vi "Init FPGA code.vi"(8 "error in (no error)":errorcluster, 11 "Device Ref in":T1 format="%.0x") -> (0 "Error out":errorcluster, 1 "DMA FIFO ref":refnum<k20>, 2 "Bitfile ref":refnum<k20>, 3 "Device Ref out":T1 format="%.0x")   [LabVIEW 2014, in "SLSC configuration Engine.lvlib"]
uses:
  SLSC configuration Engine.lvlib
  <vilib>/NI Veristand/Custom Device API/Custom Device Item Ref.ctl
  Shared/Type Defs/Device Settings.ctl
  <vilib>/NI/LVFPGA Adv Session Resources/OpenByNameSubVI.vi
  Shared/Constants.vi
  <vilib>/NI Veristand/Custom Device API/Get Item Property (Variant).vi
  <vilib>/FPGAPlugInAG/Dynamic/niLvFpga_Run_Dynamic.vi
  <vilib>/rvi/interface/common/dynamic/niFpgaEscapeDelimiterAndNull.vi
  <vilib>/Utility/error.llb/Error Cluster From Error Code.vi
  <vilib>/rvi/errors/niLvFpgaAdjustHostInterfaceError.vi
  <vilib>/rvi/interface/nirviMethod/nirviMethod.xnode
  <vilib>/NI/LVFPGA Adv Session Resources/OpenByName.xnode
  <vilib>/rvi/interface/nirviReadWriteControl/nirviReadWriteControl.xnode
  <vilib>/NI Veristand/Custom Device API/Custom Device API.lvlib
  Shared/SLSC configuration Shared.lvlib
  <vilib>/NI/LVFPGA Adv Session Resources/LVFPGAAdvSessionResources.lvlib
  NiFpgaLv.dll
  <vilib>/rvi/interface/Simulation/niFpgaSimulationCallBeginRW.vi
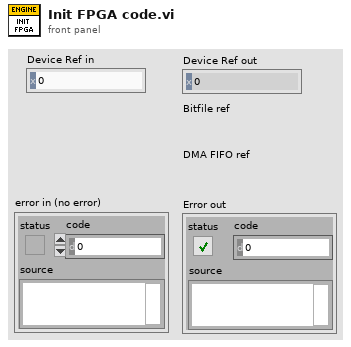
[diagram p1: front panel]
types:
  T1 = typedef "Custom Device API.lvlib/Custom Device Item Ref.ctl" = u64
  T2 = cluster{"Divide Value":u8, "Transfer Length (bits)":u8, "CS Asserted Polarity":bool, "Clock Polarity (CPOL)":bool, "Clock Phase (CPHA)":bool, "Lengthen MISO Setup":bool, "Direction Change Bit":u8, "MOSI Starts as Output":bool, "Tristatable MOSI":bool}
  T3 = typedef "SLSC configuration Shared.lvlib/Device Settings.ctl" = cluster{"RIO Address":string, "Bitfile Path":path, "Load Delay (ms)":u32, "Divide Value":u8, "Sample Rate (S/s)":u32}
  T4 = cluster{"Name":string, "Depth":u32, "Write? (Deprecated:Use Implementation)":bool, "Physical Channel":u32, "Base Address":u32, "Data Width":u32, "Data Type":enum32{"Boolean", "I8", "I16", "I32", "I64", "U8", "U16", "U32", "U64", "FXP", "CustomControl", "SGL"}, "FXP Properties":variant, "Write Window Address":u32, "Implementation":enum16{"niFpgaTargetToHost", "niFpgaHostToTarget", "niFpgaPeerToPeerWriter", "niFpgaPeerToPeerReader", "niCoreTargetToHost", "niCoreHostToTarget"}, "Control Set":u32}[]
  T5 = cluster{"Name":string, "type":variant, "indicator?":bool}[]
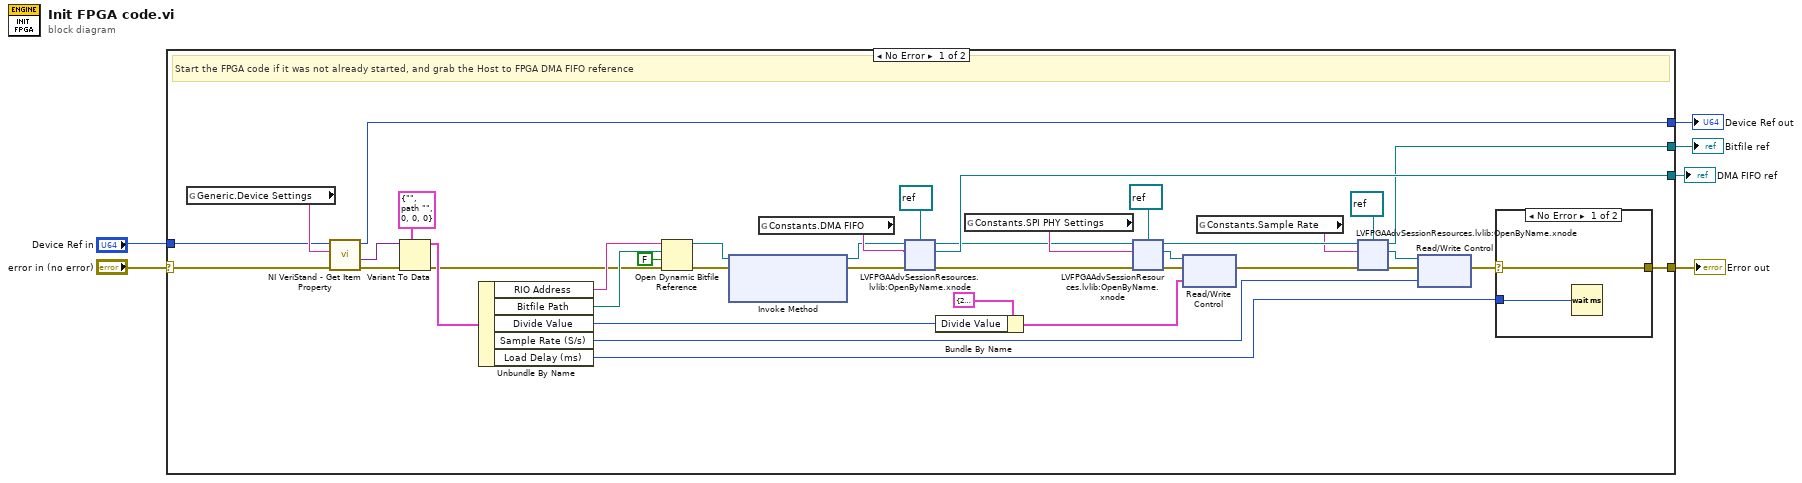
[diagram p0: block diagram]
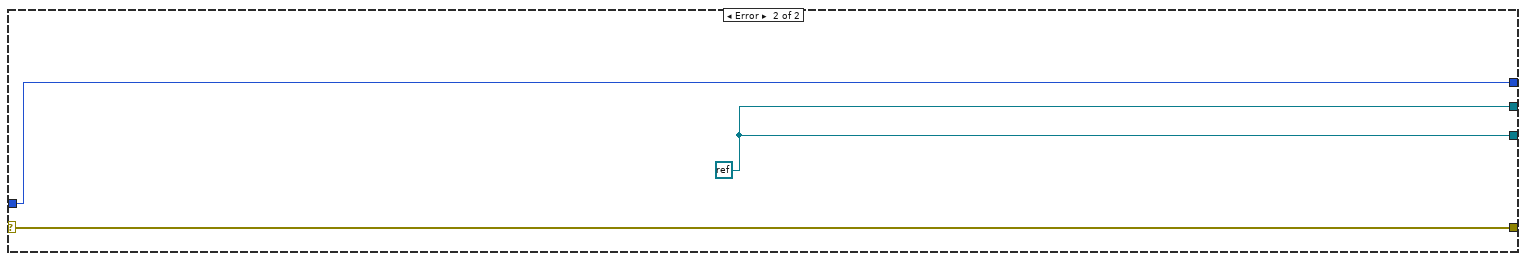
[diagram p3: hidden frame]
diagram:
  n1 = case shown="No Error" "error in (no error)" {
    selector: "error in (no error)" -> [w35 w89]
    tunnel: "Device Ref in" -> [w42 w88]
    tunnel: [w10 w90] -> w6
    tunnel: [w39 w90] -> w1
    tunnel: [w13 w89] -> w5
    tunnel: [w8 w88] -> w2
    frame No Error {
      # "Start the FPGA code if it was not already started, and grab the Host to FPGA DMA FIFO reference"
      n2 = global read "Constants.vi" "Generic.Device Settings"() -> (w43:string)
      n3 = call-poly <vilib>:"NI VeriStand - Get Item Property.vi"("error in (no error)"=w35, "Property Name"=w43, "Item Ref in"=w42) -> ("error out"=w33:errorcluster, "Value"=w34:variant, "Item Ref out"=w8:T1)  [unwired: 5 in, 1 out]
      n4 = Variant To Data(error in=w33, type=T3 {"RIO Address"="", "Bitfile Path"=path "", "Load Delay (ms)"=0, "Divide Value"=0, "Sample Rate (S/s)"=0} ("Cluster"), Variant=w34) -> (data=w31:T3, error out=w29:errorcluster)
      n5 = Unbundle By Name(w31) -> ("RIO Address"=w30:string, "Bitfile Path"=w44:path, "Divide Value"=w18:u8, "Sample Rate (S/s)"=w16:u32, "Load Delay (ms)"=w15:u32)
      n6 = Open Dynamic Bitfile Reference(0:w30, 1:w44, 2:FALSE ("Run When Loaded"), 3:w29) -> (5:w38:refnum<k20>, 8:w40:errorcluster)  [unwired: 1 in]
      n7 = xnode "Invoke Method"("FPGA VI Reference In"=w38, "error in"=w40) -> ("FPGA VI Reference Out"=w37:refnum<k20>, "error out"=w36:errorcluster)  [unwired: 1 in]
      n8 = global read "Constants.vi" "Constants.DMA FIFO"() -> (w41:string)
      n9 = xnode "LVFPGAAdvSessionResources.lvlib:OpenByName.xnode"("FPGA VI Reference in"=w37, "Resource name in"=w41, "Single resource reference type in"=refnum<k20> refnum ("Single resource reference out"), "Error in"=w36) -> ("Single resource reference out"=w39:refnum<k20>, "Error out"=w20:errorcluster, "FPGA VI Reference out"=w11:refnum<k20>)
      n10 = Bundle By Name(cluster=T2 {"Divide Value"=255, "Transfer Length (bits)"=32, "CS Asserted Polarity"=FALSE, "Clock Polarity (CPOL)"=FALSE, "Clock Phase (CPHA)"=FALSE, "Lengthen MISO Setup"=FALSE, "Direction Change Bit"=0, "MOSI Starts as Output"=FALSE, "Tristatable MOSI"=FALSE} ("SPI PHY Settings"), "Divide Value"=w18) -> (w17:T2)
      n11 = global read "Constants.vi" "Constants.SPI PHY Settings"() -> (w12:string)
      n12 = xnode "LVFPGAAdvSessionResources.lvlib:OpenByName.xnode"("FPGA VI Reference in"=w11, "Resource name in"=w12, "Single resource reference type in"=refnum<k20> refnum, "Error in"=w20) -> ("Single resource reference out"=w28:refnum<k20>, "Error out"=w27:errorcluster, "FPGA VI Reference out"=w25:refnum<k20>)
      n13 = xnode "Read/Write Control"("FPGA VI Reference In"=w28, "error in"=w27, "Value"=w17) -> ("error out"=w26:errorcluster)  [unwired: 1 out]
      n14 = global read "Constants.vi" "Constants.Sample Rate"() -> (w9:string)
      n15 = xnode "LVFPGAAdvSessionResources.lvlib:OpenByName.xnode"("FPGA VI Reference in"=w25, "Resource name in"=w9, "Single resource reference type in"=refnum<k20> refnum, "Error in"=w26) -> ("Single resource reference out"=w23:refnum<k20>, "Error out"=w24:errorcluster, "FPGA VI Reference out"=w10:refnum<k20>)
      n16 = xnode "Read/Write Control"("FPGA VI Reference In"=w23, "error in"=w24, "Value"=w16) -> ("error out"=w14:errorcluster)  [unwired: 1 out]
      n17 = case shown="No Error" w14 {
        selector: w14 -> [w46 w48]
        tunnel: w15 -> [w47 _]
        tunnel: [w46 w48] -> w13
        frame No Error {
          n18 = Wait (ms)(milliseconds to wait=w47) -> ()  [unwired: 1 out]
        }
        frame Error {
        }
      }
    }
    frame Error {
      w90 = refnum<k0> refnum
    }
  }
  "Bitfile ref" <- w6
  "Error out" <- w5
  "Device Ref out" <- w2
  "DMA FIFO ref" <- w1
